vi "init server.vi"(8 "error in (no error)":errorcluster, 11 "Header content in":refnum<class "Header content.lvclass">) -> (0 "error out":errorcluster, 3 "Header content out":refnum<class "Header content.lvclass">)   [LabVIEW 2018, in "Header content.lvclass"]
uses:
  Header content.lvclass
  Server/Server.lvclass
  Server/Server.lvclass/Server.ctl
  Header content.lvclass/Header content.ctl
panel:
  in  "Server.lvclass":refnum<class "Server.lvclass">
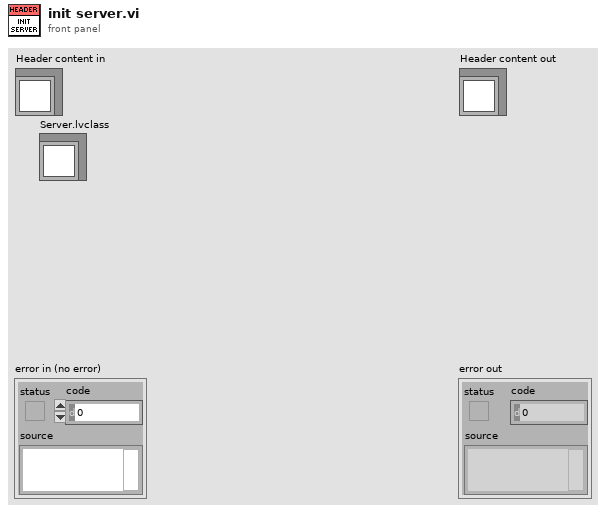
[diagram p1: front panel]
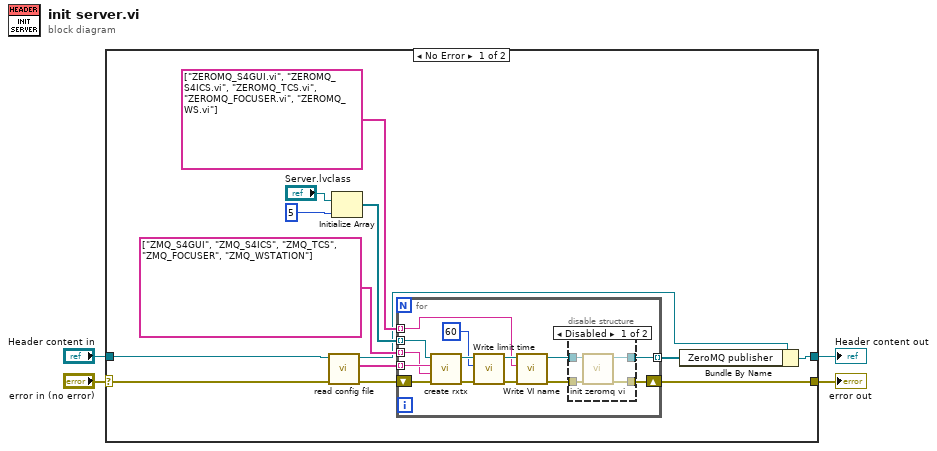
[diagram p0: block diagram]
diagram:
  n1 = case shown="No Error" "error in (no error)" {
    selector: "error in (no error)" -> [w10 w39]
    tunnel: [w17 w39] -> w3
    tunnel: [w16 w38] -> w1
    tunnel: "Header content in" -> [w6 w38]
    frame No Error {
      n2 = call "read config file.vi"("error in (no error)"=w10, "Header content in"=w6) -> ("error out"=w9:errorcluster, "remote IPs"=w8:string[], "Header content out"=w5:refnum<class "Header content.lvclass">)  [unwired: 7 in]
      n3 = Initialize Array("Server.lvclass", 5 ("dimension size")) -> (w15:refnum<class "Server.lvclass">[])
      n4 = for {
        shift-right: [w19] -> w17
        shift-left: w9 -> [w31]
        tunnel: w8 -> [w27] mode=indexing
        tunnel: w15 -> [w29] mode=indexing
        tunnel: [w20] -> w13 mode=indexing
        tunnel: string[] ["ZMQ_S4GUI", "ZMQ_S4ICS", "ZMQ_TCS", "ZMQ_FOCUSER", "ZMQ_WSTATION"] -> [w25] mode=indexing
        tunnel: string[] ["ZEROMQ_S4GUI.vi", "ZEROMQ_S4ICS.vi", "ZEROMQ_TCS.vi", "ZEROMQ_FOCUSER.vi", "ZEROMQ_WS.vi"] -> [w18] mode=indexing
        n5 = call "create rxtx.vi"("error in (no error)"=w31, "qeue name"=w25, "remote IP"=w27, "Server in"=w29) -> ("error out"=w30:errorcluster, "Server out"=w28:refnum<class "Server.lvclass">)  [unwired: 6 in]
        n6 = call "Write limit time.vi"("error in (no error)"=w30, "limit time"=u16 60, "Server in"=w28) -> ("error out"=w22:errorcluster, "Server out"=w21:refnum<class "Server.lvclass">)  [unwired: 7 in]
        n7 = call "Write VI name.vi"("error in (no error)"=w22, "VI name"=w18, "Server in"=w21) -> ("error out"=w23:errorcluster, "Server out"=w24:refnum<class "Server.lvclass">)  [unwired: 7 in]
        n8 = disable-structure shown="Disabled" {
          disable-tunnel: w24 -> [w35 w37]
          disable-tunnel: w23 -> [w34 w36]
          disable-tunnel: [w33 w37] -> w20
          disable-tunnel: [w32 w36] -> w19
          frame Disabled {
            n9 = call "init zeromq vi.vi"("error in (no error)"=w34, "Server in"=w35) -> ("error out"=w32:errorcluster, "Server out"=w33:refnum<class "Server.lvclass">)  [unwired: 8 in]
          }
          frame Enabled {
          }
        }
      }
      n10 = Bundle By Name(cluster=w5, "ZeroMQ publisher"=w13) -> (w16:refnum<class "Header content.lvclass">)
    }
    frame Error {
    }
  }
  "error out" <- w3
  "Header content out" <- w1
